vi "指尖指中弯曲.vi"(9 "上限":dbl, 10 "指中":refnum<vi>, 11 "指尖":refnum<vi>) -> ()   [LabVIEW 2016]
uses:
  <vilib>/picture/3D Picture Control/NI_3D Picture Control.lvlib
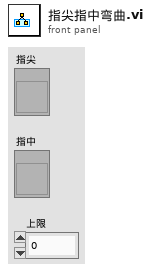
[diagram p1: front panel]
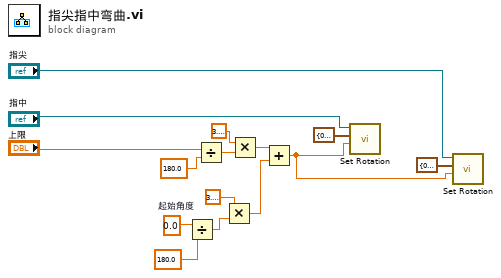
[diagram p0: block diagram]
diagram:
  w9 = 0.0  # 起始角度
  n1 = Divide(x=w9, y=180.0) -> (x/y=w11:dbl)
  n2 = Divide(x="上限", y=180.0) -> (x/y=w6:dbl)
  n3 = Multiply(x=3.141592653589793, y=w11) -> (x*y=w13:dbl)
  n4 = Multiply(x=3.141592653589793, y=w6) -> (x*y=w8:dbl)
  n5 = Add(x=w8, y=w13) -> (x+y=w15:dbl)
  n6 = call <vilib>:"Set Rotation.vi"("Angle"=w15, "Axis"=cluster{"X":sgl, "Y":sgl, "Z":sgl} {"X"=0.0, "Y"=1.0, "Z"=0.0}, "Scene Object"="指中") -> ()  [unwired: 7 in, 2 out]
  n7 = call <vilib>:"Set Rotation.vi"("Angle"=w15, "Axis"=cluster{"X":sgl, "Y":sgl, "Z":sgl} {"X"=0.0, "Y"=1.0, "Z"=0.0}, "Scene Object"="指尖") -> ()  [unwired: 7 in, 2 out]
